vi "hosts.deserialize.orderbook.commands.vi"(11 "DataIn":u64[](array[numeric]) format="%.0x") -> (3 "OrderBook.Command[]":T1[](array[typedef]))   [LabVIEW 2020]
uses:
  fpga/orderbook.command.ctl
  fpga/orderbook.command.type.ctl
  fpga/fpganow.common.fpga.lvlib
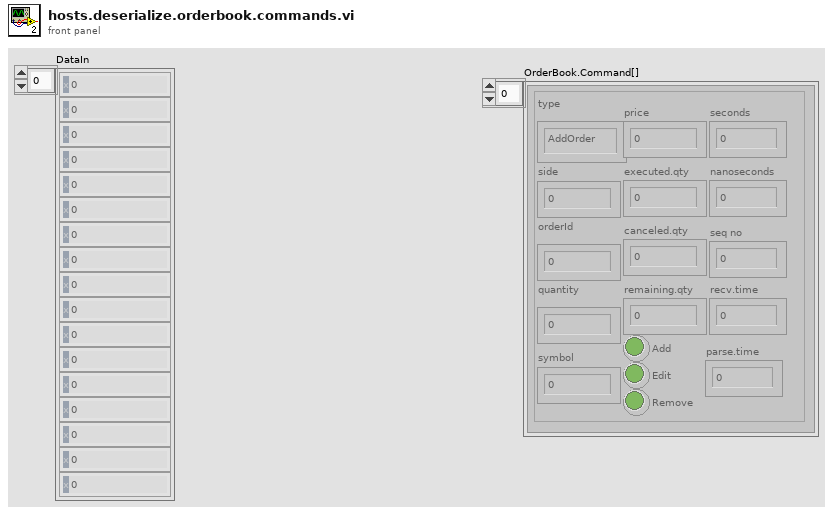
[diagram p1: front panel]
types:
  T1 = typedef "fpganow.common.fpga.lvlib/orderbook.command.ctl" = cluster{"type":T2, "side":u8, "orderId ":u64, "quantity":u32, "symbol":u64, "price":u64, "executed.qty":u32, "canceled.qty":u32, "remaining.qty":u32, "seconds":u64, "nanoseconds":u64, "Add":bool, "Edit":bool, "Remove":bool, "seq no":u32, "recv.time":u64, "parse.time":u64}
  T2 = typedef "fpganow.common.fpga.lvlib/orderbook.command.type.ctl" = enum8{"Time", "AddOrder", "OrderExecuted", "OrderExecutedAtPrice", "ReduceSize", "ModifyOrder", "DeleteOrder", "Get.Everything", "Get.All.Orders", "Get.Top"}
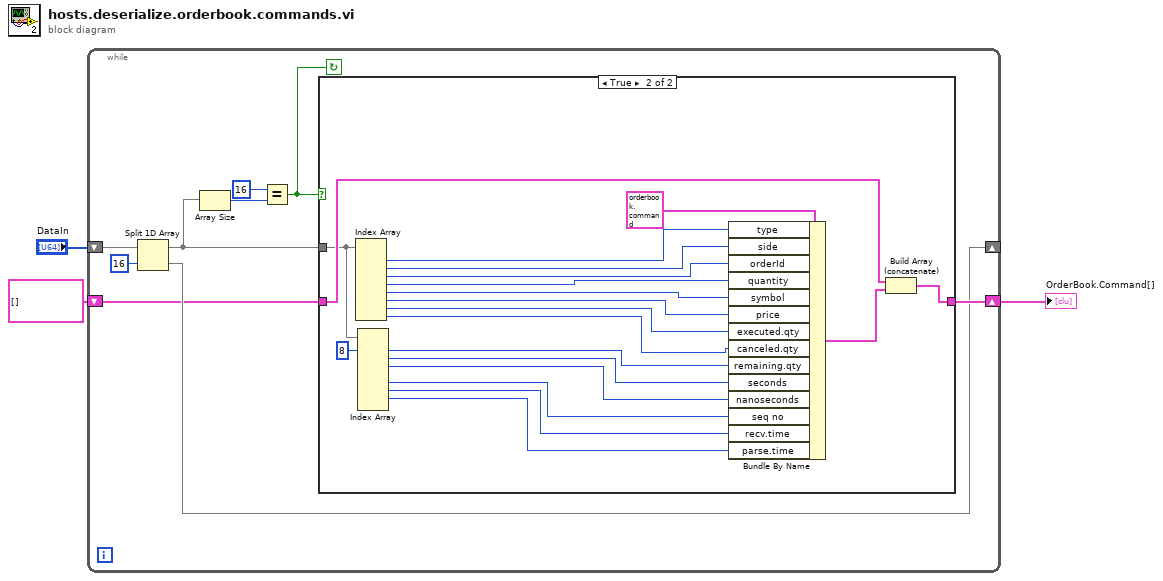
[diagram p0: block diagram]
diagram:
  n1 = while {
    shift-right: [w8] -> _
    shift-left: "DataIn" -> [w12]
    shift-right: [w10] -> w2
    shift-left: T1[] [] -> [w4]
    stop <- w5 continue-if-true
    n2 = Split 1D Array(array=w12, index=16) -> (first subarray=w9:u64[], second subarray=w8:u64[])
    n3 = Array Size(array=w9) -> (size(s)=w7:i32)
    n4 = Equal?(x=16, y=w7) -> (x = y?=w5:bool)
    n5 = case shown="True" w5 {
      tunnel: [w13 w23] -> w10
      tunnel: w9 -> [_ w21]
      tunnel: w4 -> [w13 w22]
      frame False {
      }
      frame True {
        n6 = Index Array(array=w21) -> (element #1=w32:u64, element #2=w31:u64, element #3=w30:u64, element #4=w29:u64, element #5=w28:u64, element #6=w27:u64, element #7=w26:u64, element #8=w25:u64)  [unwired: 8 in]
        n7 = Index Array(array=w21, index #1=8 ("index")) -> (element #1=w19:u64, element #2=w18:u64, element #3=w17:u64, element #5=w16:u64, element #6=w15:u64, element #7=w14:u64)  [unwired: 7 in, 2 out]
        n8 = Bundle By Name(cluster=T1 {"type"=enum."AddOrder", "side"=0, "orderId "=0, "quantity"=0, "symbol"=0, "price"=0, "executed.qty"=0, "canceled.qty"=0, "remaining.qty"=0, "seconds"=0, "nanoseconds"=0, "Add"=FALSE, "Edit"=FALSE, "Remove"=FALSE, "seq no"=0, "recv.time"=0, "parse.time"=0} ("Cluster"), "type"=w32, "side"=w31, "orderId"=w30, "quantity"=w29, "symbol"=w28, "price"=w27, "executed.qty"=w26, "canceled.qty"=w25, "remaining.qty"=w19, "seconds"=w18, "nanoseconds"=w17, "seq no"=w16, "recv.time"=w15, "parse.time"=w14) -> (w24:T1)
        n9 = Build Array (concatenate)(w22, w24) -> (w23:T1[])
      }
    }
  }
  "OrderBook.Command[]" <- w2
